vi "Set Bitmap.vi"(8 "error in (no error)":errorcluster, 10 "Bitmap":u32[][](array[numeric]), 11 "Bitmap Canvas in":refnum<class "Bitmap Canvas.lvclass">) -> (0 "error out":errorcluster, 3 "Bitmap Canvas out":refnum<class "Bitmap Canvas.lvclass">)   [LabVIEW 2020, in "Glyph Drawer.lvlib" / "Bitmap Canvas.lvclass"]
uses:
  Bitmap Canvas.lvclass
  Bitmap Canvas.lvclass/Bitmap Canvas.ctl
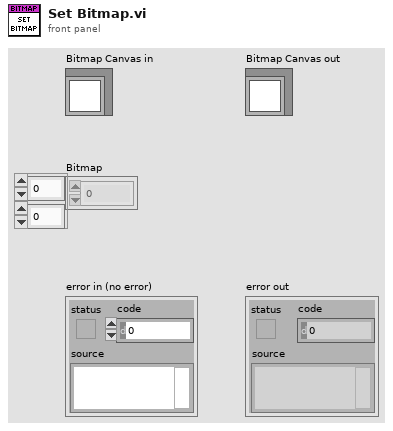
[diagram p1: front panel]
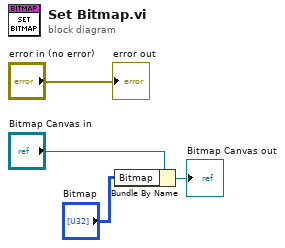
[diagram p0: block diagram]
diagram:
  n1 = Bundle By Name(cluster="Bitmap Canvas in", "Bitmap"="Bitmap") -> (→"Bitmap Canvas out":refnum<class "Bitmap Canvas.lvclass">)
  "error out" <- "error in (no error)"
